vi "Program Initialization.vi"(7 "menu reference":refnum<k9>, 8 "error in":errorcluster, 11 "classes in":T1) -> (0 "error out":errorcluster, 3 "classes out":T1)   [LabVIEW 2011]
uses:
  Controls/Class Objects.ctl
  Modules/File/Configuration/Configuration.lvclass
  Modules/Hardware/Power Supply/Power Supply.lvclass
  Modules/Hardware/Mass Flow Controller/Mass Flow Controller.lvclass
  Modules/Hardware/PID/PID.lvclass
  Modules/Hardware/Valve Controller/Valve Controller.lvclass
  Modules/Hardware/Multimeter/Multimeter.lvclass
  Modules/Hardware/Vapour Generator/Vapour Generator.lvclass
  Modules/File/TDMS/TDMS.lvclass
  Controls/User Interface Action.ctl
  Functional Global Data/Device Params Global.ctl
  Functional Global Data/Status Bar.ctl
  Functional Global Data/Globals.ctl
  Functional Global Data/Analysis Data.ctl
  Modules/Menu/Menu Action.ctl
  Functional Global Data/Run Data.ctl
  Modules/File/Configuration/File Type.ctl
  Controls/Class Labels.ctl
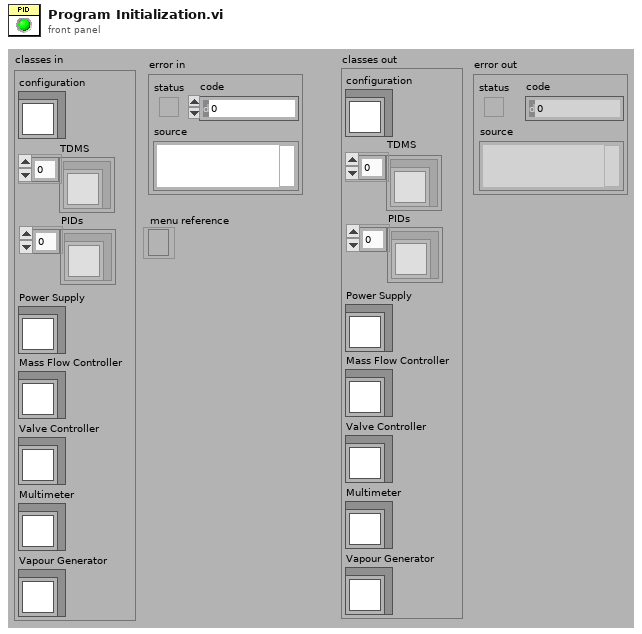
[diagram p1: front panel]
types:
  T1 = typedef "Class Objects.ctl" = cluster{"configuration":refnum<class "Configuration.lvclass">, "TDMS":refnum<class "TDMS.lvclass">[], "Power Supply":refnum<class "Power Supply.lvclass">, "Mass Flow Controller":refnum<class "Mass Flow Controller.lvclass">, "Valve Controller":refnum<class "Valve Controller.lvclass">, "Multimeter":refnum<class "Multimeter.lvclass">, "Vapour Generator":refnum<class "Vapour Generator.lvclass">, "PIDs":refnum<class "PID.lvclass">[]}
  T2 = typedef "User Interface Action.ctl" = enum16{"Initialize", "Data Acquisition Disable", "Data View Disable", "Sample Set", "Sample Set 2D Data", "Sample Set x0 & dx", "Sample Add", "Sample Set Cursor", "Sample Set Offset & Multiplier", "Sample Set Axis Labels", "Sample Parameters Disabled", "Sample Parameters Update", "Run Update", "Run Set Offset & Multiplier", "Run Set Axis Labels", "Run Set Cursor", "Run Set Disabled", "Run Parameters Update", "Run Parameters Disabled", "Run Number Set", "Run Number Set Range", "Run Number Set Disabled", "Sample Number Set", "Sample Number Set Range", "Notes Set Value", "Update Plot", "Set Plot Parameters", "Update Concentration Plot", "Time Set", "Clear DAQ Display", "Clear Analysis Display", "Status Bar Set", "Progress Bar Set", "Display Mode Set", "Experiment Type Set", "Analysis Plot Average Set", "Stop"}
  T3 = enum8{"Enabled", "Disabled", "Disabled and Grayed Out"}
  T4 = typedef "Device Params Global.ctl" = enum16{"Initialize", "Get Device Settings", "Get Device Connections", "Set Device Settings", "Set Device Connections", "Get All Device Properties"}
  T5 = typedef "Status Bar.ctl" = enum16{"Insert Into Status Bar", "Get Status Bar", "Initialize"}
  T6 = typedef "Globals.ctl" = enum16{"Initialize", "Get DAQ Params", "Get Data Display Params", "Set DAQ Params", "Set Data Display Params"}
  T7 = typedef "Analysis Data.ctl" = enum16{"Initialize", "Add Plot", "Get Plots"}
  T8 = typedef "Menu Action.ctl" = enum16{"Initialize", "Insert Item", "Remove Item", "Set Checked Item", "Get Checked Item", "Get Item Index", "Item Present?", "Stop"}
  T9 = typedef "Run Data.ctl" = enum16{"Initialize", "Add Sample Channel", "Set Run", "Get Number of Runs", "Set Run Params", "Get Spectrum", "Get Run Params", "Get Sample Params", "Get History", "Get Averaged History", "Get Run Param Names", "Set Run Param Names", "Get Sample Param Names", "Set Sample Param Names", "Get MFC Flow Rate Challenge Profile", "Get History Average"}
  T10 = typedef "Configuration.lvclass/File Type.ctl" = enum16{"INI", "XML"}
  T11 = typedef "Class Labels.ctl" = enum16{"Configuration", "TDMS", "PID", "Power Supply", "Vapour Generator", "MFC", "NMR", "Valve Controller", "Multimeter"}
  T12 = typedef "Device Connections.ctl" = cluster{"Detector":cluster{"Detector Type":T13, "Connection":bool, "B-M PID":T14, "INL PID Connections":T15}, "Power Supply":cluster{"Type":enum16{"Stanford Research PS350", "Keithley 2400"}, "Connection":bool, "VISA resource name":refnum<visa-resource-name>}, "Mass Flow Controller":cluster{"Type":enum16{"Aalborg GFC17"}, "Connection":bool, "Aalborg GFC17":T17}, "Valve Controller":cluster{"Type":T18, "Connection":bool, "SMC - INL":cluster{"VISA resource name":refnum<visa-resource-name>}}, "Multimeter":cluster{"Multimeter Type":T19, "Connection":bool, "VISA resource name":refnum<visa-resource-name>}, "Vapour Generator":cluster{"Type":T20, "Connection":bool, "Owlstone Gen-SYS":T21}}
  T13 = typedef "Detector Type.ctl" = enum16{"INL PID", "Baseline-Mocon piD-TECH plus"}
  T14 = typedef "Baseline Mocon piD-Tech plus.lvclass/Connections.ctl" = cluster{"AI DAQmx channel":tag}
  T15 = typedef "INL PID Connections.ctl" = cluster{"PIDs":u8, "Integrator DAQ Channels 1":T16, "Integrator DAQ Channels 2":T16}
  T16 = typedef "INL PID.lvclass/Integrator DAQmx Channels.ctl" = cluster{"V0":tag, "S1":tag, "S2":tag}
  T17 = typedef "Aalborg GFC17.lvclass/Aalborg GFC17 Connections.ctl" = cluster{"flow rate setpoint channel":tag, "flow rate reading channel":tag, "valve channel":tag}
  T18 = typedef "Valve Type.ctl" = enum16{"SMC - INL"}
  T19 = typedef "Multimeter Type.ctl" = enum16{"Agilent 3458A"}
  T20 = typedef "Vapour Generator Type.ctl" = enum16{"Owlstone GEN-SYS"}
  T21 = typedef "Owlstone GEN-SYS.lvclass/GEN-SYS Connections.ctl" = cluster{"GEN-SYS VISA resource name":refnum<visa-resource-name>, "OVG-4":cluster{"Flow Address":u8, "Temp Address":u8}, "OHG-4":cluster{"Flow Address":u8, "Easydew VISA resource name":refnum<visa-resource-name>}}
  T22 = typedef "Data Acquisition Parameters.ctl" = cluster{"Experiment Type":T23, "Experiment Name":string, "Operator Name":string, "Notes":string, "TDMS File Path":path, "Data Acquisition State":bool, "PID Voltage Sweep":T24, "MFC Challenge Profile - Heaviside Step":T25, "MFC Challenge Profile":T26, "MFC Challenge Profile - Staircase":T27}
  T23 = typedef "DAQ Type.ctl" = enum16{"PID Sample", "PID with PS Challenge", "PID with MFC Challenge", "Multimeter Sample", "Multimeter with MFC Challenge"}
  T24 = typedef "PID Voltage Seep Settings.ctl" = cluster{"Voltage Step (V)":dbl, "Voltage Range (V)":cluster{u16, u16}, "Time Step (s)":dbl, "Voltage Step Direction":enum16{"High 2 Low", "Low 2 High"}}
  T25 = typedef "MFC Challenge Profile - Heaviside Step.ctl" = cluster{"Valve Open Duration":u16, "MFC Flow Rate":dbl, "Valve Open Repeats":u16, "Valve Open Start":u16}
  T26 = typedef "MFC Challen Profile Type.ctl" = enum16{"Heaviside", "Staircase"}
  T27 = typedef "MFC Challenge Profile - Staircase.ctl" = cluster{"Step Time Duration":u16, "Step Flow Rate":dbl, "Steps":u16, "Valve Open Start":u16, "Recovery":bool, "Repeats":u16}
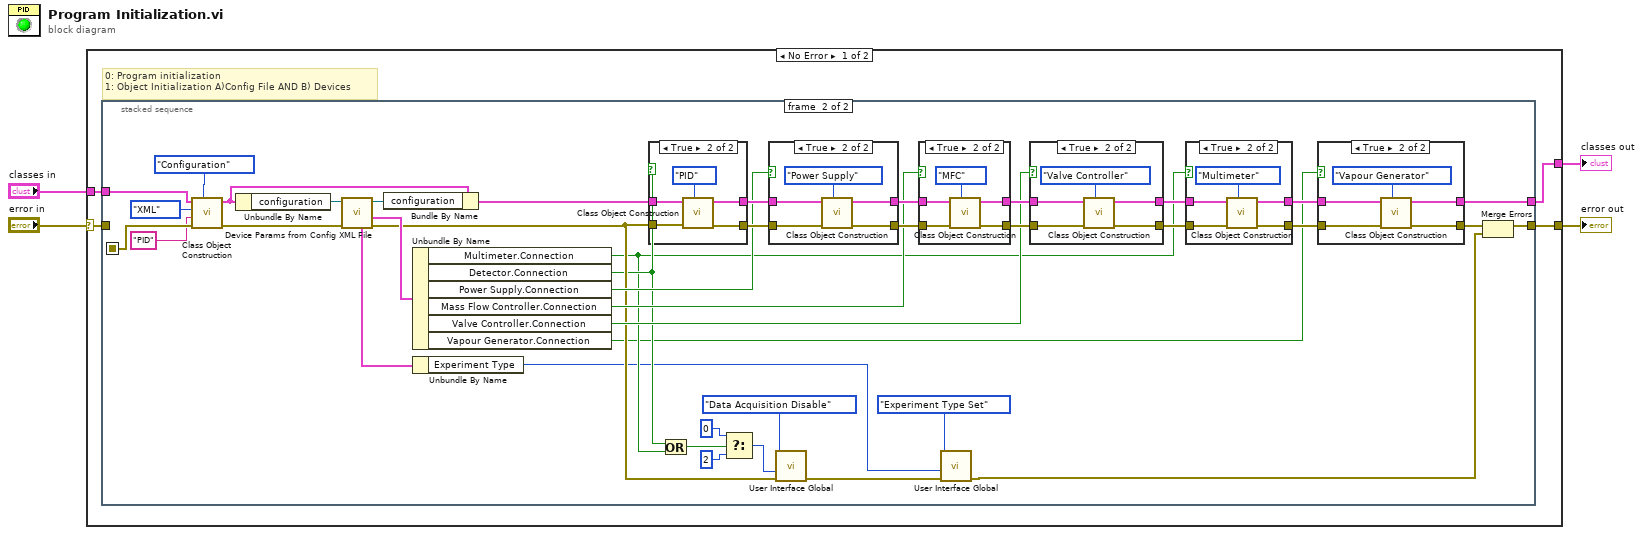
[diagram p0: block diagram]
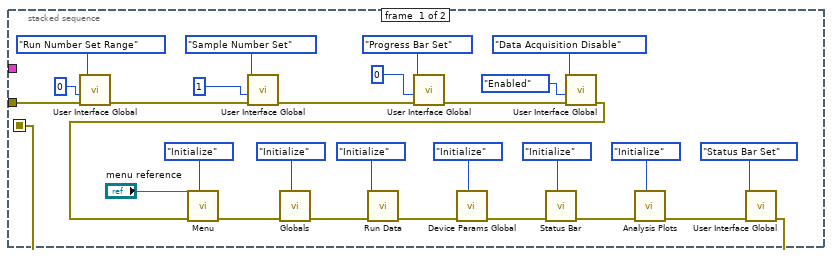
[diagram p2: hidden frame]
diagram:
  n1 = case shown="No Error" "error in" {
    selector: "error in" -> [w8 w121]
    tunnel: [w7 w121] -> w3
    tunnel: "classes in" -> [w6 w120]
    tunnel: [w5 w120] -> w1
    frame No Error {
      # "0: Program initialization\n1: Object Initialization A)Config File AND B) Devices"
      n2 = stacked-sequence {
        seq-local: [w9 _] -> [_ w76]
        tunnel: w8 -> [w24 _]
        tunnel: [_ w60] -> w7
        tunnel: w6 -> [_ w53]
        tunnel: [_ w44] -> w5
        frame #0 {
          n3 = call "User Interface Global.vi"("error in"=w24, "data1"=u16 0 ("Run"), "action"=User_Interface_Action."Run Number Set Range") -> ("error out"=w30:errorcluster)  [unwired: 8 in]
          n4 = call "User Interface Global.vi"("error in"=w30, "data1"=u32 1 ("Run"), "action"=User_Interface_Action."Sample Number Set") -> ("error out"=w13:errorcluster)  [unwired: 8 in]
          n5 = call "User Interface Global.vi"("error in"=w13, "data1"=u8 0, "action"=User_Interface_Action."Progress Bar Set") -> ("error out"=w11:errorcluster)  [unwired: 8 in]
          n6 = call "User Interface Global.vi"("error in"=w11, "data1"=T3."Enabled" ("Disabled"), "action"=User_Interface_Action."Data Acquisition Disable") -> ("error out"=w10:errorcluster)  [unwired: 8 in]
          n7 = call "Menu.vi"("action"=Menu_Action."Initialize" ("Menu"), "error in"=w10, "menu reference"="menu reference") -> ("error out"=w22:errorcluster)  [unwired: 5 in, 3 out]
          n8 = call "Globals.vi"("action"=Globals."Initialize", "error in"=w22) -> ("error out"=w21:errorcluster)  [unwired: 7 in, 2 out]
          n9 = call "Run Data.vi"("error in"=w21, "action"=Run_Data."Initialize" ("Action")) -> ("error out"=w20:errorcluster)  [unwired: 6 in, 3 out]
          n10 = call "Device Params Global.vi"("action"=Device_Params_Global."Initialize", "error in"=w20) -> ("error out"=w19:errorcluster)  [unwired: 7 in, 2 out]
          n11 = call "Status Bar.vi"("action"=Status_Bar."Initialize", "error in"=w19) -> ("error out"=w18:errorcluster)  [unwired: 8 in, 1 out]
          n12 = call "Analysis Plots.vi"("action"=Analysis_Data."Initialize", "error in"=w18) -> ("error out"=w17:errorcluster)  [unwired: 7 in, 2 out]
          n13 = call "User Interface Global.vi"("error in"=w17, "action"=User_Interface_Action."Status Bar Set" ("Action")) -> ("error out"=w9:errorcluster)  [unwired: 9 in]
        }
        frame #1 {
          n14 = call "Class Object Construction.vi"("class"=Class_Labels."Configuration" ("Enum"), "error in"=w76, "param2"="PID", "param 1"=File_Type."XML" ("File Type"), "classes in"=w53) -> ("error out"=w70:errorcluster, "classes out"=w71:T1)  [unwired: 4 in]
          n15 = Unbundle By Name(w71) -> ("configuration"=w72:refnum<class "Configuration.lvclass">)
          n16 = call "Device Params from Config XML File.vi"("error in"=w70, "Configuration in"=w72) -> ("error out"=w50:errorcluster, "Device Connections"=w57:T12, "Configuration out"=w73:refnum<class "Configuration.lvclass">, "Data Acquisition"=w41:T22)  [unwired: 5 in, 1 out]
          n17 = Bundle By Name(cluster=w71, "configuration"=w73) -> (w65:T1)
          n18 = Unbundle By Name(w57) -> ("Multimeter.Connection"=w48:bool, "Detector.Connection"=w49:bool, "Power Supply.Connection"=w56:bool, "Mass Flow Controller.Connection"=w55:bool, "Valve Controller.Connection"=w54:bool, "Vapour Generator.Connection"=w42:bool)
          n19 = Unbundle By Name(w41) -> ("Experiment Type"=w39:T23)
          n20 = case shown="True" w49 {
            tunnel: w65 -> [w114 w118]
            tunnel: [w114 w117] -> w66
            tunnel: w50 -> [w113 w116]
            tunnel: [w113 w115] -> w67
            frame False {
            }
            frame True {
              n21 = call "Class Object Construction.vi"("class"=Class_Labels."PID" ("Class"), "error in"=w116, "classes in"=w118) -> ("error out"=w115:errorcluster, "classes out"=w117:T1)  [unwired: 6 in]
            }
          }
          n22 = Or(x=w49, y=w48) -> (x .or. y?=w47:bool)
          n23 = Select(t=0, s=w47, f=2) -> (s? t:f=w61:i32)
          n24 = case shown="True" w56 {
            tunnel: w66 -> [w107 w111]
            tunnel: w67 -> [w106 w110]
            tunnel: [w107 w109] -> w68
            tunnel: [w106 w108] -> w69
            frame False {
            }
            frame True {
              n25 = call "Class Object Construction.vi"("class"=Class_Labels."Power Supply" ("Class"), "error in"=w110, "classes in"=w111) -> ("error out"=w108:errorcluster, "classes out"=w109:T1)  [unwired: 6 in]
            }
          }
          n26 = call "User Interface Global.vi"("error in"=w50, "data1"=w61, "action"=User_Interface_Action."Data Acquisition Disable") -> ("error out"=w38:errorcluster)  [unwired: 8 in]
          n27 = case shown="True" w55 {
            tunnel: w68 -> [w100 w104]
            tunnel: w69 -> [w99 w103]
            tunnel: [w100 w102] -> w58
            tunnel: [w99 w101] -> w59
            frame False {
            }
            frame True {
              n28 = call "Class Object Construction.vi"("class"=Class_Labels."MFC" ("Class"), "error in"=w103, "classes in"=w104) -> ("error out"=w101:errorcluster, "classes out"=w102:T1)  [unwired: 6 in]
            }
          }
          n29 = call "User Interface Global.vi"("error in"=w38, "data1"=w39, "action"=User_Interface_Action."Experiment Type Set") -> ("error out"=w37:errorcluster)  [unwired: 8 in]
          n30 = case shown="True" w54 {
            tunnel: w58 -> [w93 w97]
            tunnel: w59 -> [w92 w96]
            tunnel: [w93 w95] -> w52
            tunnel: [w92 w94] -> w51
            frame False {
            }
            frame True {
              n31 = call "Class Object Construction.vi"("class"=Class_Labels."Valve Controller" ("Class"), "error in"=w96, "classes in"=w97) -> ("error out"=w94:errorcluster, "classes out"=w95:T1)  [unwired: 6 in]
            }
          }
          n32 = case shown="True" w48 {
            tunnel: w52 -> [w86 w90]
            tunnel: w51 -> [w85 w89]
            tunnel: [w86 w88] -> w45
            tunnel: [w85 w87] -> w46
            frame False {
            }
            frame True {
              n33 = call "Class Object Construction.vi"("class"=Class_Labels."Multimeter" ("Class"), "error in"=w89, "classes in"=w90) -> ("error out"=w87:errorcluster, "classes out"=w88:T1)  [unwired: 6 in]
            }
          }
          n34 = case shown="True" w42 {
            tunnel: w45 -> [w79 w83]
            tunnel: w46 -> [w78 w82]
            tunnel: [w79 w81] -> w44
            tunnel: [w78 w80] -> w43
            frame False {
            }
            frame True {
              n35 = call "Class Object Construction.vi"("class"=Class_Labels."Vapour Generator" ("Class"), "error in"=w82, "classes in"=w83) -> ("error out"=w80:errorcluster, "classes out"=w81:T1)  [unwired: 6 in]
            }
          }
          n36 = Merge Errors(w43, w37) -> (w60:errorcluster)
        }
      }
    }
    frame Error {
    }
  }
  "error out" <- w3
  "classes out" <- w1
